vi "PL Open.vi"(8 "error in":errorcluster) -> (0 "error out":errorcluster, 1 "Notifiers":T2, 2 "Queues":T1, 3 "User Event":refnum<user-event>, 5 "Event Registration Refnum":refnum<event-registration>)   [LabVIEW 2015]
doc: "Creates and initializes main application resources (notifiers, queues, user events etc.)"
uses:
  Notifiers/Notifiers.ctl
  Message Queue/All Message Queues.ctl
  Message Queue/Message Cluster.ctl
  Message Queue/Message Queue.lvlib
  User Event - EHL Stop/User Event - EHL Stop.lvlib
  Notifiers/Notifiers.lvlib
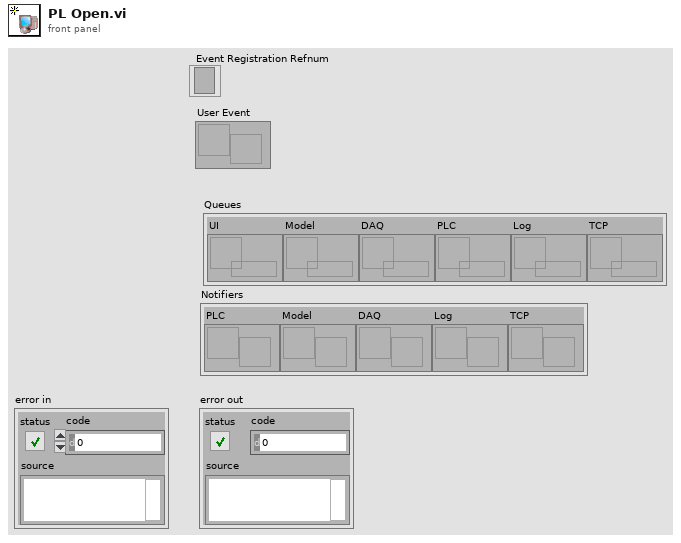
[diagram p1: front panel]
types:
  T1 = typedef "Message Queue.lvlib/All Message Queues.ctl" = cluster{"UI":refnum<queue>, "Model":refnum<queue>, "DAQ":refnum<queue>, "PLC":refnum<queue>, "Log":refnum<queue>, "TCP":refnum<queue>}
  T2 = typedef "Notifiers.lvlib/Notifiers.ctl" = cluster{"PLC":refnum<notifier>, "Model":refnum<notifier>, "DAQ":refnum<notifier>, "Log":refnum<notifier>, "TCP":refnum<notifier>}
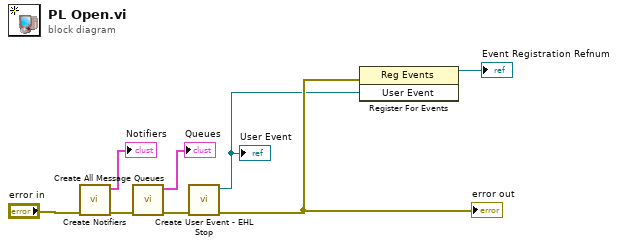
[diagram p0: block diagram]
diagram:
  n1 = call "Create Notifiers.vi"("error in"="error in") -> ("error out"=w4:errorcluster, "Notifiers"=→"Notifiers":T2)  [unwired: 9 in]
  n2 = call "Create All Message Queues.vi"("error in"=w4) -> ("error out"=w6:errorcluster, "Queues"=→"Queues":T1)  [unwired: 9 in]
  n3 = call "Create User Event - EHL Stop.vi"("error in"=w6) -> ("error out"=w3:errorcluster, "User Event"=w2:refnum<user-event>)  [unwired: 9 in]
  "error out" <- w3
  "User Event" <- w2
  n4 = register-events(error in=w3, w2) -> (reference out=→"Event Registration Refnum":refnum<event-registration>)  [unwired: 1 in, 1 out]
